vi "channel modify.vi"() -> (2 "changes match?":bool)   [LabVIEW 2013, in "Shared Memory Tests.lvlib"]
uses:
  Shared Memory Tests.lvlib
  module/configuration/Shared Memory Configuration.lvclass
  <vilib>/NI/Tag Bus/tag/tag descriptor.lvclass
  <vilib>/NI/Tag Bus Module Framework/channel/TBM channel.lvclass
  module/configuration/line configuration.ctl
  <vilib>/NI/Tag Bus/tag/Data Type.ctl
panel:
  out "modified data type":T1
  out "data type":T1
  out "modified name":string
  out "name":string
  out "modified tag":T2[](array[typedef])
  out "original tag":T2[](array[typedef])
  out "error out":errorcluster
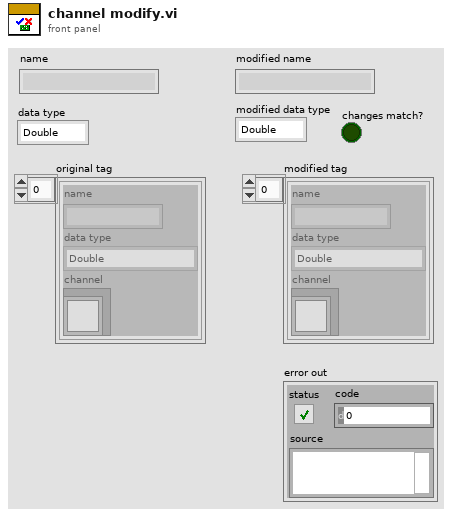
[diagram p1: front panel]
types:
  T1 = typedef "tag bus.lvlib/tag descriptor.lvclass/Data Type.ctl" = enum16{"Double", "Single", "I64", "I32", "I16", "I8", "U64", "U32", "U16", "U8", "Boolean", "String", "Array of Double", "Array of Single", "Array of I64", "Array of I32", "Array of I16", "Array of I8", "Array of U64", "Array of U32", "Array of U16", "Array of U8", "Array of Boolean", "Array of String"}
  T2 = typedef "Shared Memory Configuration.lvclass/line configuration.ctl" = cluster{"name":string, "data type":T1, "channel":refnum<class "TBM channel.lvclass">}
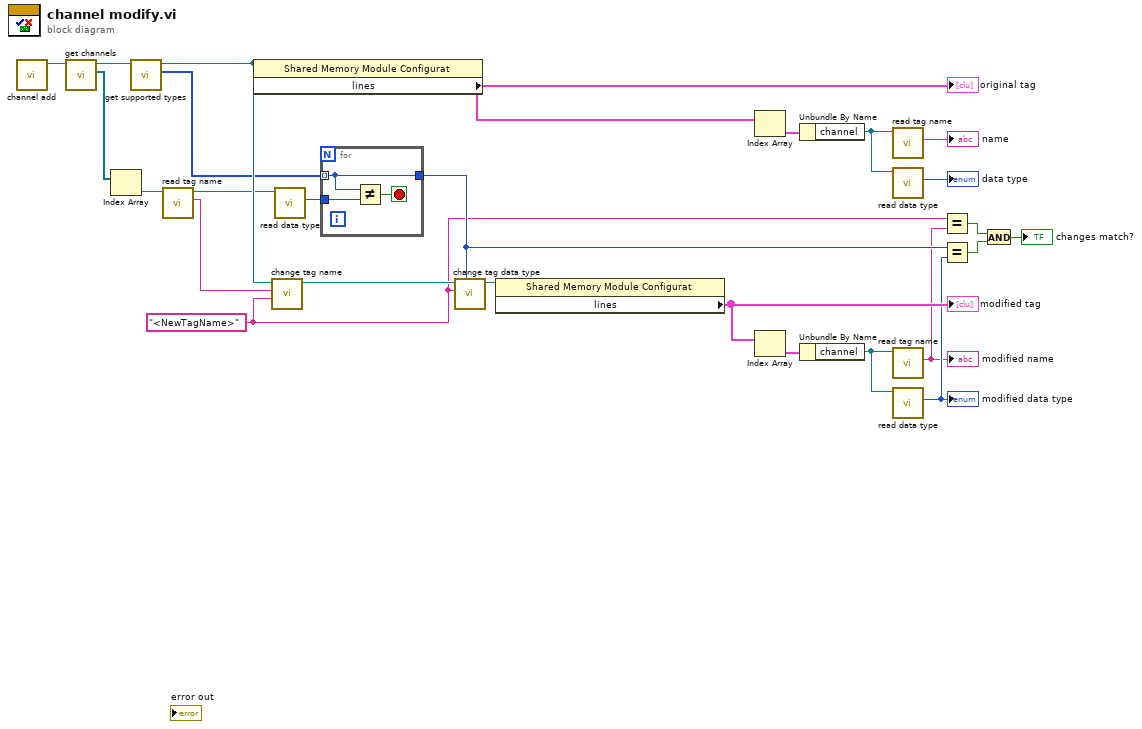
[diagram p0: block diagram]
diagram:
  w5 = "<NewTagName>"
  n1 = call "channel add.vi"() -> ("configuration out"=w18:refnum<class "Shared Memory Configuration.lvclass">)  [unwired: 7 in, 4 out]
  n2 = call-dynamic "get channels.vi"("shared memory module configuration"=w18) -> ("channels"=w17:refnum<class "TBM channel.lvclass">[], "shared memory module configuration out"=w14:refnum<class "Shared Memory Configuration.lvclass">)  [unwired: 9 in]
  n3 = Index Array(array=w17) -> (element=w16:refnum<class "TBM channel.lvclass">)  [unwired: 1 in]
  n4 = call-dynamic "get supported types.vi"("shared memory module configuration"=w14) -> ("supported types"=w11:T1[], "shared memory module configuration out"=w13:refnum<class "Shared Memory Configuration.lvclass">)  [unwired: 8 in, 1 out]
  n5 = call <vilib>:"read tag name.vi"("system tag in"=w16) -> ("name"=w15:string, "system tag out"=w12:refnum<class "TBM channel.lvclass">)  [unwired: 8 in, 1 out]
  n6 = property class="Shared Memory Module Configurat"(reference=w13) -> ("lines"=w26:T2[])  [unwired: 1 in, 2 out]
  "original tag" <- w26
  n7 = call "change tag name.vi"("new name"=w5, "old name"=w15, "shared memory module configuration"=w13) -> ("shared memory module configuration out"=w10:refnum<class "Shared Memory Configuration.lvclass">)  [unwired: 5 in, 3 out]
  n8 = call <vilib>:"read data type.vi"("system tag in"=w12) -> ("data type"=w8:T1)  [unwired: 8 in, 2 out]
  n9 = for {
    tunnel: w11 -> [w28] mode=indexing
    tunnel: w8 -> [w29]
    tunnel: [w28] -> w7
    stop <- w27 stop-if-true
    n10 = Not Equal?(x=w28, y=w29) -> (x != y?=w27:bool)
  }
  n11 = call "change tag data type.vi"("data type"=w7, "tag name"=w5, "shared memory module configuration in"=w10) -> ("shared memory module configuration out"=w9:refnum<class "Shared Memory Configuration.lvclass">)  [unwired: 6 in, 2 out]
  n12 = property class="Shared Memory Module Configurat"(reference=w9) -> ("lines"=w22:T2[])  [unwired: 1 in, 2 out]
  "modified tag" <- w22
  n13 = Index Array(array=w26) -> (element=w25:T2)  [unwired: 1 in]
  n14 = Index Array(array=w22) -> (element=w23:T2)  [unwired: 1 in]
  n15 = Unbundle By Name(w25) -> ("channel"=w20:refnum<class "TBM channel.lvclass">)
  n16 = Unbundle By Name(w23) -> ("channel"=w19:refnum<class "TBM channel.lvclass">)
  n17 = call <vilib>:"read tag name.vi"("system tag in"=w20) -> ("name"=→"name":string)  [unwired: 8 in, 2 out]
  n18 = call <vilib>:"read data type.vi"("system tag in"=w20) -> ("data type"=→"data type":T1)  [unwired: 8 in, 2 out]
  n19 = call <vilib>:"read tag name.vi"("system tag in"=w19) -> ("name"=w4:string)  [unwired: 8 in, 2 out]
  "modified name" <- w4
  n20 = call <vilib>:"read data type.vi"("system tag in"=w19) -> ("data type"=w6:T1)  [unwired: 8 in, 2 out]
  "modified data type" <- w6
  n21 = Equal?(x=w5, y=w4) -> (x = y?=w3:bool)
  n22 = Equal?(x=w7, y=w6) -> (x = y?=w2:bool)
  n23 = And(x=w3, y=w2) -> (x .and. y?=→"changes match?":bool)
